vi "Set to PWM.vi"(11 "Raw in":dbl[](array[numeric])) -> (2 "Scaled out 2":u32, 3 "Scaled out 1":u32)   [LabVIEW 2011]
uses:
  MyGlobal.vi
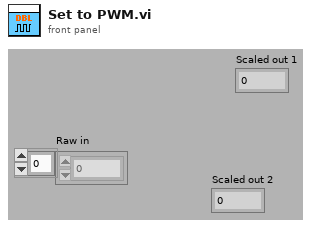
[diagram p1: front panel]
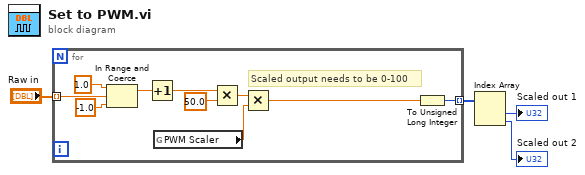
[diagram p0: block diagram]
diagram:
  n1 = for {
    tunnel: [w6] -> w3 mode=indexing
    tunnel: "Raw in" -> [w5] mode=indexing
    # "Scaled output needs to be 0-100"
    n2 = In Range and Coerce(upper limit=1.0, x=w5, lower limit=-1.0) -> (coerced(x)=w12:dbl)  [unwired: 1 out]
    n3 = Increment(x=w12) -> (x+1=w11:dbl)
    n4 = global read "MyGlobal.vi" "PWM Scaler"() -> (w8:dbl)
    n5 = Multiply(x=w11, y=50.0) -> (x*y=w9:dbl)
    n6 = Multiply(x=w9, y=w8) -> (x*y=w7:dbl)
    n7 = To Unsigned Long Integer(number=w7) -> (unsigned 32bit integer=w6:u32)
  }
  n8 = Index Array(array=w3) -> (element #1=→"Scaled out 1":u32, element #2=→"Scaled out 2":u32)  [unwired: 2 in]
